vi "practica2_ejercicio1.vi"() -> ()   [LabVIEW 2011]
panel:
  out "FACTORIAL":i32
  out "MENSAJE":string
  in  "Numeric":dbl
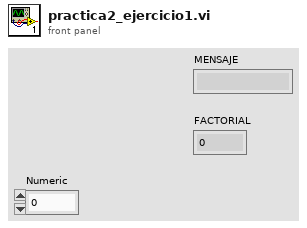
[diagram p1: front panel]
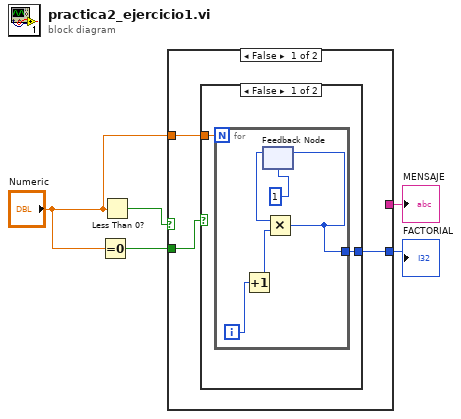
[diagram p0: block diagram]
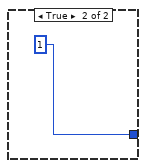
[diagram p2: hidden frame]
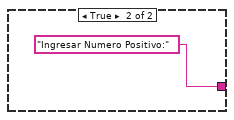
[diagram p3: hidden frame]
diagram:
  n1 = Equal To 0?(x="Numeric") -> (x = 0?=w3:bool)
  n2 = Less Than 0?(x="Numeric") -> (x < 0?=w5:bool)
  n3 = case shown="False" w5 {
    tunnel: [_ "Ingresar Numero Positivo:"] -> w4
    tunnel: w3 -> [w8 _]
    tunnel: [w7 _] -> w2
    tunnel: "Numeric" -> [w6 _]
    frame False {
      n4 = case shown="False" w8 {
        tunnel: [w10 1] -> w7
        tunnel: w6 -> [w9 _]
        frame False {
          n5 = for {
            N: w9 -> [_]
            tunnel: [w11] -> w10
            i -> [w15]
            n6 = Increment(x=w15) -> (x+1=w14:i32)
            n7 = feedback #1(1) -> (w12:i32)
            n8 = Multiply(x=w12, y=w14) -> (x*y=w11:i32)
            n9 = feedback-in #1(w11) -> ()
          }
        }
        frame True {
        }
      }
    }
    frame True {
    }
  }
  "MENSAJE" <- w4
  "FACTORIAL" <- w2
